vi "Read drive.vi"(8 "error in (no error)":errorcluster, 11 "PAS Data in":refnum<class "PAS Data.lvclass">) -> (0 "error out":errorcluster, 2 "drive":bool, 3 "PAS Data out":refnum<class "PAS Data.lvclass">)   [LabVIEW 2018, in "PAS Library.lvlib" / "PAS Data.lvclass"]
uses:
  PAS Data.lvclass
  PAS Data.lvclass/PAS Data.ctl
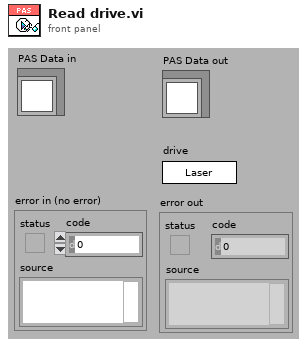
[diagram p1: front panel]
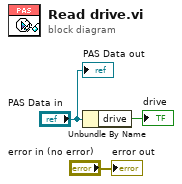
[diagram p0: block diagram]
diagram:
  n1 = Unbundle By Name("PAS Data in") -> ("drive"=→"drive":bool)
  "error out" <- "error in (no error)"
  "PAS Data out" <- "PAS Data in"
